vi "Robot Systems.vi"(11 "Robot Commands":T1) -> ()   [LabVIEW 2014]
uses:
  Joystick/Robot Commands.ctl
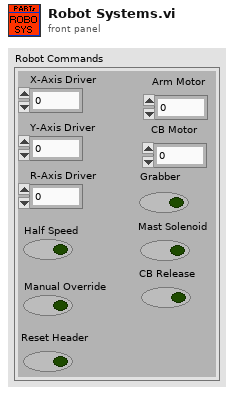
[diagram p1: front panel]
types:
  T1 = typedef "Robot Commands.ctl" = cluster{"X-Axis Driver":dbl, "Y-Axis Driver":dbl, "R-Axis Driver":dbl, "Half Speed":bool, "Manual Override":bool, "Reset Header":bool, "Arm Motor":dbl, "CB Motor":dbl, "Grabber":bool, "Mast Solenoid":bool, "CB Release":bool}
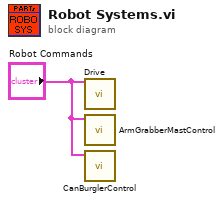
[diagram p0: block diagram]
diagram:
  n1 = call "Drive.vi"("Robot Commands"="Robot Commands") -> ()  [unwired: 14 in, 1 out]
  n2 = call "ArmGrabberMastControl.vi"("Robot Commands"="Robot Commands") -> ()  [unwired: 10 in, 1 out]
  n3 = call "CanBurglerControl.vi"("Robot Commands"="Robot Commands") -> ()  [unwired: 10 in, 1 out]
